vi "encodeStream.vi"(8 "error in (no error)":errorcluster, 11 "tBSONObjectID in":refnum<class "tBSONObjectID.lvclass">) -> (0 "error out":errorcluster, 2 "Byte Array":u8[](array[numeric]), 3 "tBSONObjectID out":refnum<class "tBSONObjectID.lvclass">)   [LabVIEW 2013, in "BSON.lvlib" / "tBSONObjectID.lvclass"]
uses:
  tBSONObjectID.lvclass
  tBSONElement/tBSONElement.lvclass
  tBSONObjectID.lvclass/tBSONObjectID.ctl
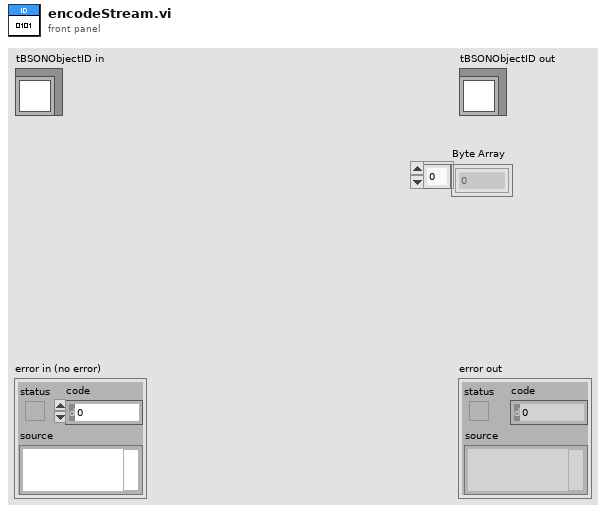
[diagram p1: front panel]
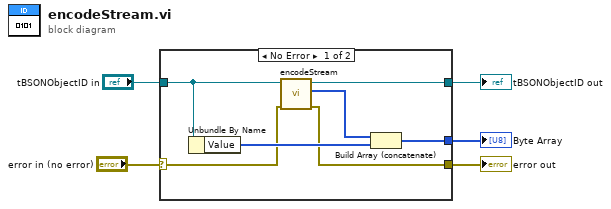
[diagram p0: block diagram]
diagram:
  n1 = case shown="No Error" "error in (no error)" {
    selector: "error in (no error)" -> [w9 w13]
    tunnel: "tBSONObjectID in" -> [w10 w14]
    tunnel: [w6 w14] -> w4
    tunnel: [w8 w13] -> w2
    tunnel: [w12 _] -> w3
    frame No Error {
      n2 = Unbundle By Name(w10) -> ("Value"=w11:u8[])
      n3 = call-parent "encodeStream.vi"("error in (no error)"=w9, "tBSONElement in"=w10) -> ("error out"=w8:errorcluster, "Byte Array"=w7:u8[], "tBSONElement out"=w6:refnum<class "tBSONObjectID.lvclass">)  [unwired: 7 in]
      n4 = Build Array (concatenate)(w7, w11) -> (w12:u8[])
    }
    frame Error {
    }
  }
  "error out" <- w2
  "tBSONObjectID out" <- w4
  "Byte Array" <- w3
